vi "Rename Options to Flags.vi"(1 "Options":T1={"Atomic"=FALSE, "Native"=FALSE, "Overwrite"=TRUE}) -> (0 "Flags":i32)   [LabVIEW 2021, in "Field_RnD_Services_LIBSSH2_Toolkit.lvlib" / "SFTP.lvclass"]
doc: "Converts Rename options to an integer bit flag value."
uses:
  SFTP.lvclass
  Type Definitions/Rename Options.ctl
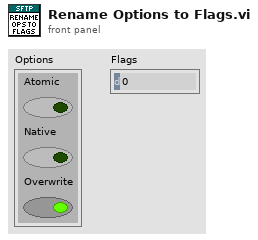
[diagram p1: front panel]
types:
  T1 = typedef "Field_RnD_Services_LIBSSH2_Toolkit.lvlib/SFTP.lvclass/Rename Options.ctl" = cluster{"Atomic":bool, "Native":bool, "Overwrite":bool}
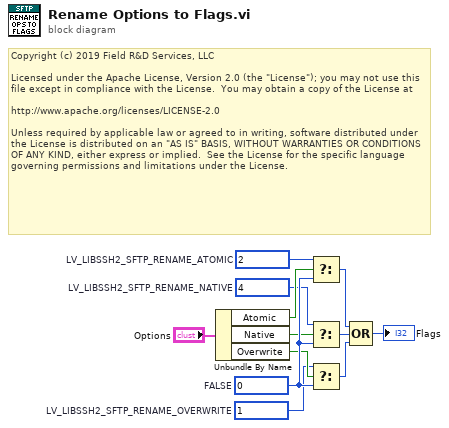
[diagram p0: block diagram]
diagram:
  w1 = 1  # LV_LIBSSH2_SFTP_RENAME_OVERWRITE
  w2 = 4  # LV_LIBSSH2_SFTP_RENAME_NATIVE
  w3 = 2  # LV_LIBSSH2_SFTP_RENAME_ATOMIC
  w12 = 0  # FALSE
  # "Copyright (c) 2019 Field R&D Services, LLC\n\nLicensed under the Apache License, Version 2.0 (the \"License\"); you may not use this file except in compliance with the License.  You may obtain a copy of the License at\n\nhttp://www.apache.org/licenses/LICENSE-2.0\n\nUnless required by applicable law or agreed to in writing, software distributed under the License is distributed on an \"AS IS\" BASIS, WITHOUT WARRANTIES OR CONDITIONS OF ANY KIND, either express or implied.  See the License for the specific language governing permissions and limitations under the License."
  n1 = Unbundle By Name("Options") -> ("Atomic"=w4:bool, "Native"=w5:bool, "Overwrite"=w6:bool)
  n2 = Select(t=w3, s=w4, f=w12) -> (s? t:f=w11:i32)
  n3 = Select(t=w2, s=w5, f=w12) -> (s? t:f=w10:i32)
  n4 = Select(t=w1, s=w6, f=w12) -> (s? t:f=w9:i32)
  n5 = Compound Arithmetic op=OR(w11, w10, w9) -> (→"Flags":i32)
